vi "DecodeNumericValue.vi"(10 "DataLen":i32, 11 "Frame":string) -> (1 "NumericValue":u32, 3 "Remainder":string)   [LabVIEW 2016]
doc: "Split Frame into Numeric Hex String and Suffix using DataLen. Return converted NumericValue and Suffix."
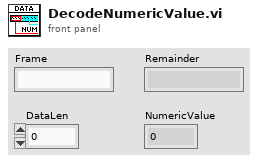
[diagram p1: front panel]
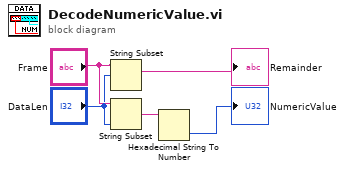
[diagram p0: block diagram]
diagram:
  n1 = String Subset(string="Frame", offset (0)="DataLen") -> (substring=→"Remainder":string)  [unwired: 1 in]
  n2 = String Subset(string="Frame", length (rest)="DataLen") -> (substring=w4:string)  [unwired: 1 in]
  n3 = Hexadecimal String To Number(string=w4) -> (number=→"NumericValue":u32)  [unwired: 2 in, 1 out]
